vi "LoggingMessageLoop.vi"(8 "Error In":errorcluster, 11 "CommunicationRefs":T1) -> (0 "Error Out":errorcluster)   [LabVIEW 2015]
uses:
  TypeDefs/CommunicationRefs.ctl
  TypeDefs/MessageCluster.ctl
  TypeDefs/FlowData.ctl
  TypeDefs/ClsLastSample.ctl
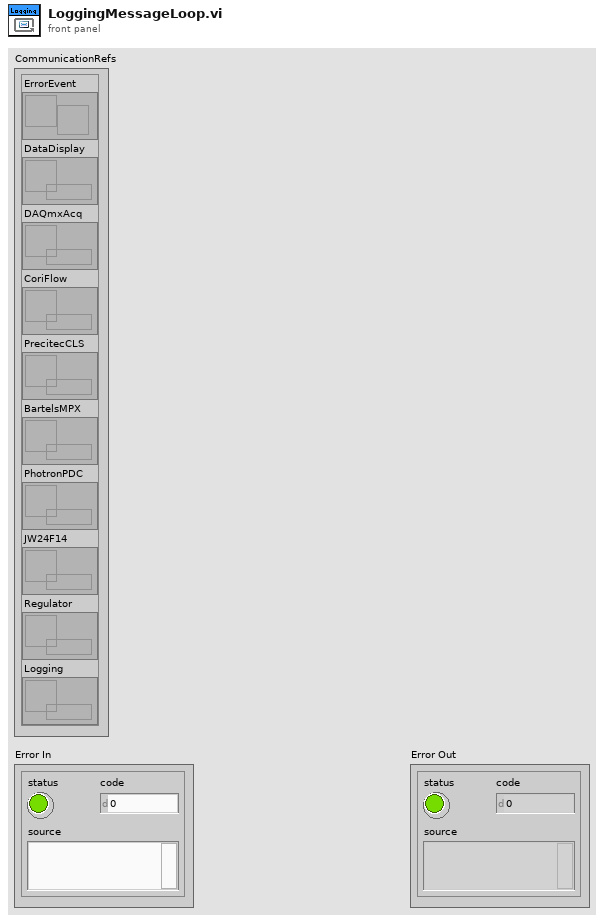
[diagram p1: front panel]
types:
  T1 = typedef "CommunicationRefs.ctl" = cluster{"ErrorEvent":refnum<user-event>, "DataDisplay":refnum<queue>, "DAQmxAcq":refnum<queue>, "CoriFlow":refnum<queue>, "PrecitecCLS":refnum<queue>, "BartelsMPX":refnum<queue>, "PhotronPDC":refnum<queue>, "JW24F14":refnum<queue>, "Regulator":refnum<queue>, "Logging":refnum<queue>}
  T2 = enum16{"open", "open or create", "create or replace", "create", "open (read-only)"}
  T3 = typedef "FlowData.ctl" = cluster{"Setpoint Direct":sgl, "Setpoint Percentage":dbl, "Flow Direct":sgl, "Flow Percentage [%]":dbl, "Fluid Temperature [°C]":sgl, "Fluid Density [kg/m³]":sgl, "Alarm":string}
  T4 = typedef "ClsLastSample.ctl" = cluster{"Global Signals":dbl[], "Peak Signals":dbl[][], "Film Height [µm]":dbl, "standard deviation [µm]":dbl, "variance":dbl}
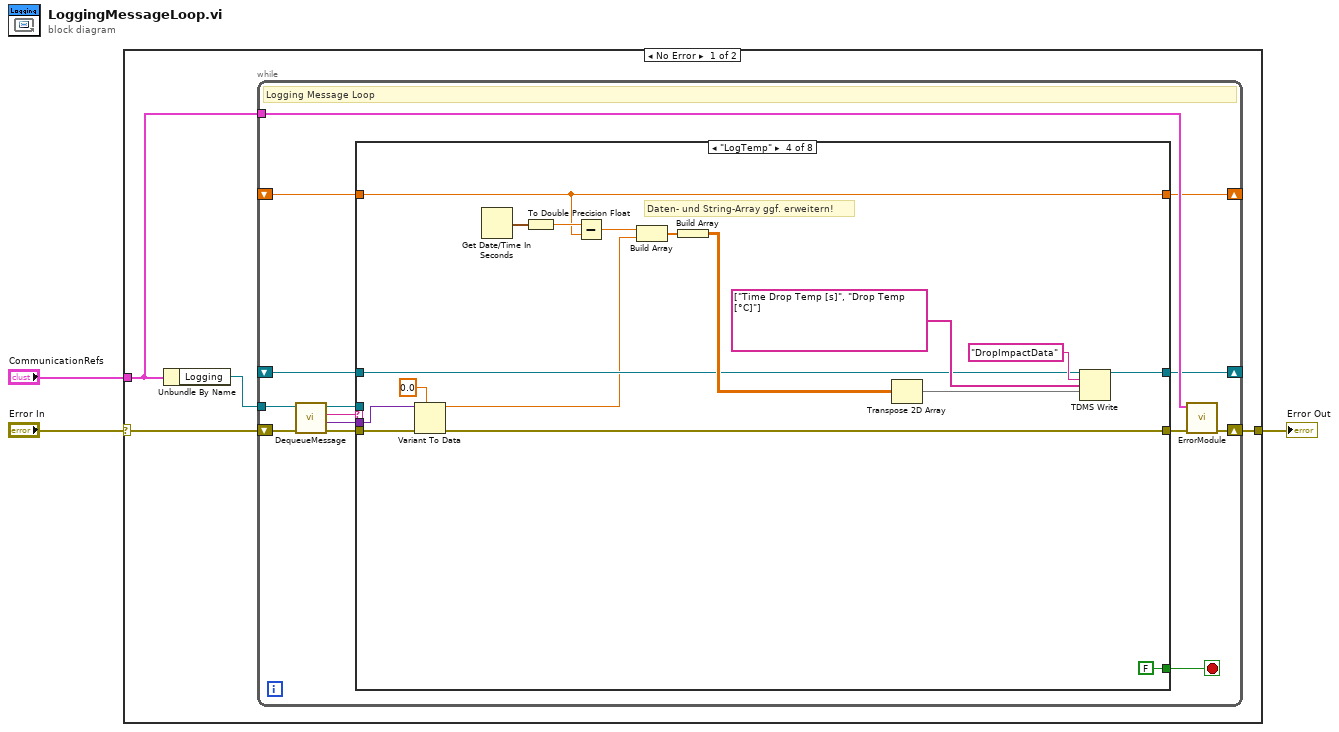
[diagram p0: block diagram]
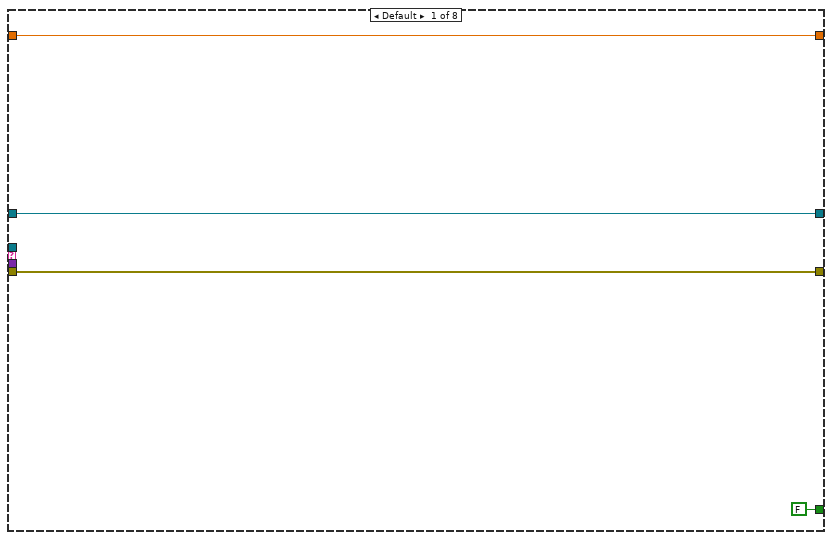
[diagram p2: hidden frame]
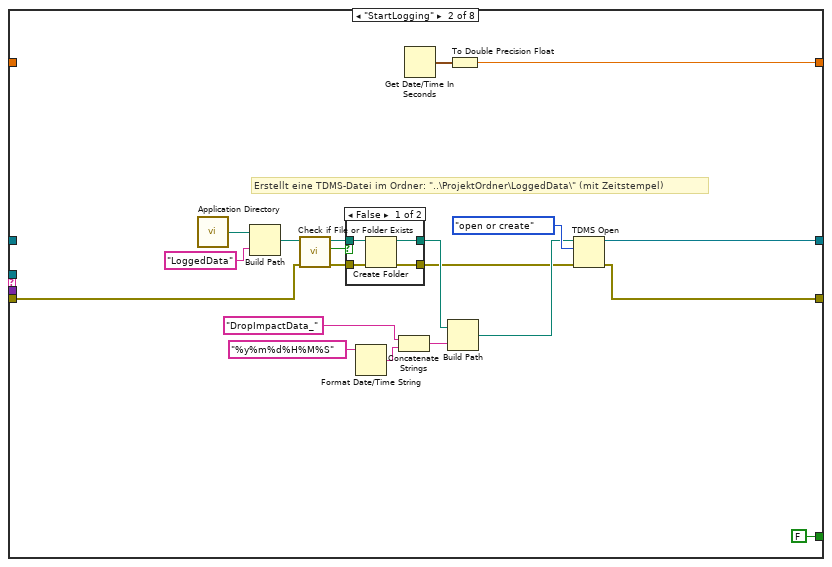
[diagram p3: hidden frame]
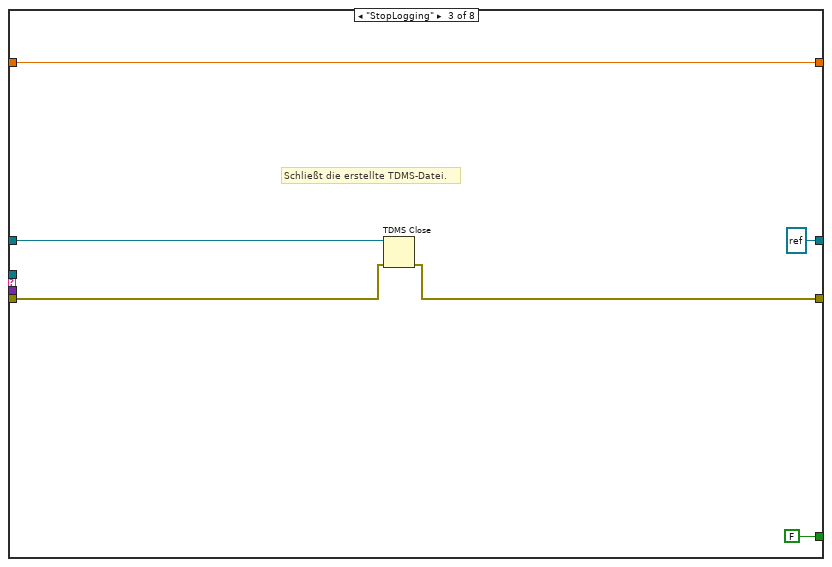
[diagram p5: hidden frame]
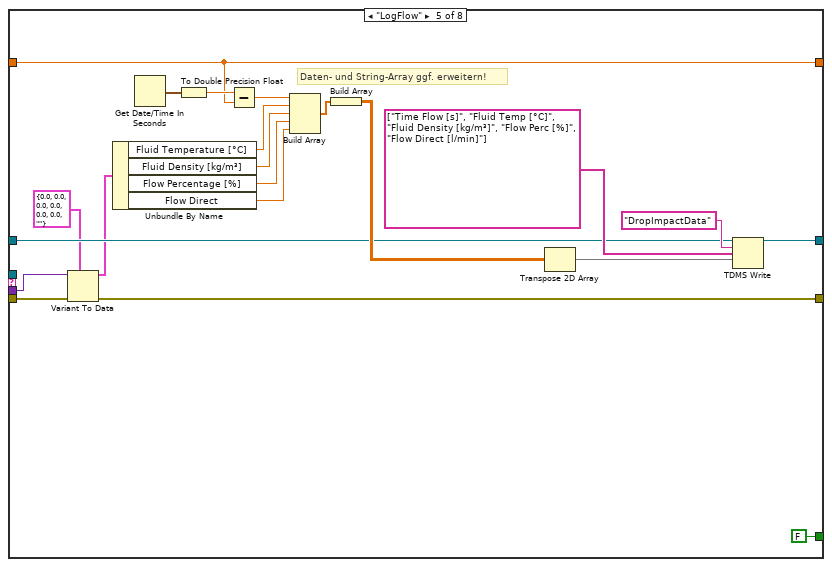
[diagram p6: hidden frame]
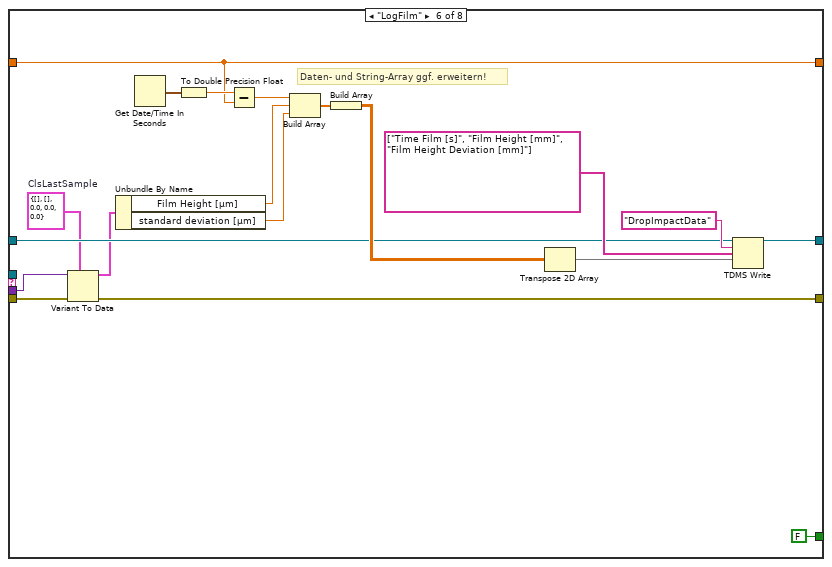
[diagram p7: hidden frame]
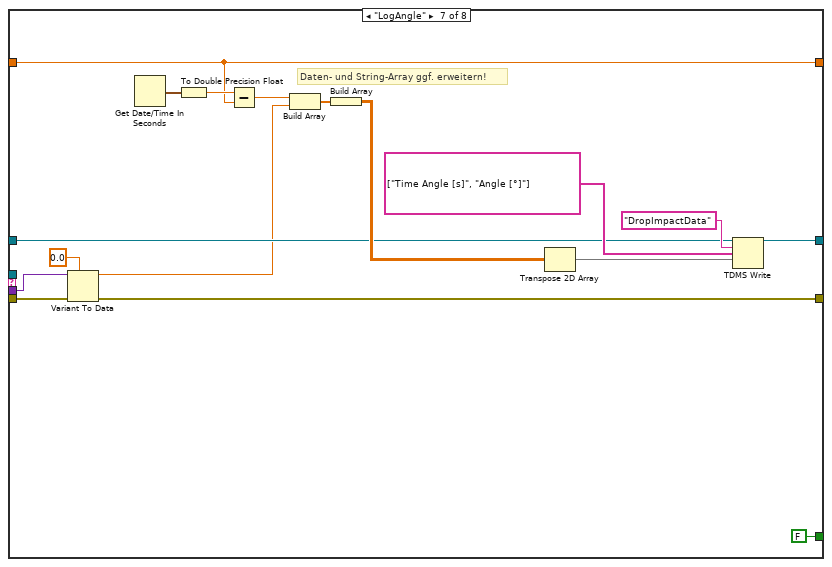
[diagram p8: hidden frame]
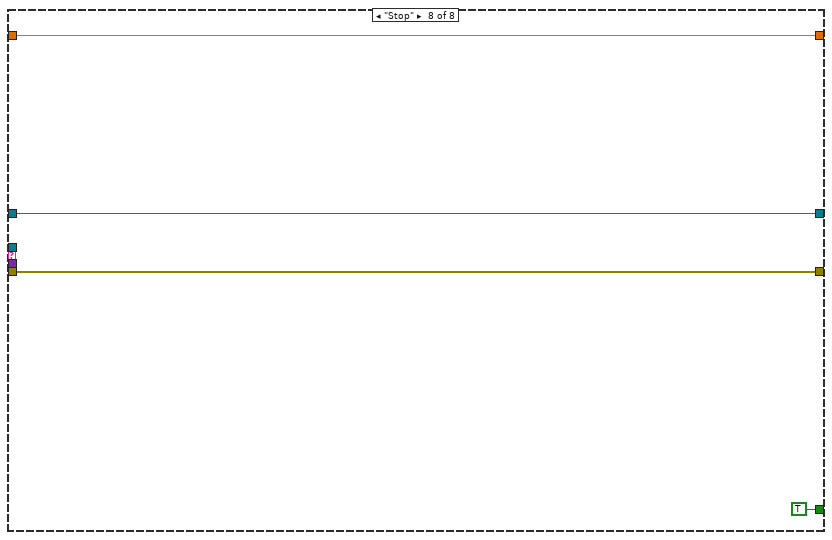
[diagram p9: hidden frame]
diagram:
  n1 = case shown="No Error" "Error In" {
    selector: "Error In" -> [w6 w136]
    tunnel: [w5 w136] -> w2
    tunnel: "CommunicationRefs" -> [w4 _]
    frame No Error {
      n2 = Unbundle By Name(w4) -> ("Logging"=w7:refnum<queue>)
      n3 = while {
        tunnel: w7 -> [w21]
        tunnel: w4 -> [w14]
        shift-right: [w15] -> w5
        shift-left: w6 -> [w20]
        shift-right: [w11] -> _
        shift-left: _ -> [w10]
        shift-right: [w9] -> _
        shift-left: _ -> [w8]
        stop <- w13 stop-if-true
        # "Logging Message Loop"
        n4 = call "DequeueMessage.vi"("error in (no error)"=w20, "MessageQueue"=w21) -> ("error out"=w16:errorcluster, "MessageData"=w17:variant, "Message"=w18:string, "dupMessageQueue"=w19:refnum<queue>)  [unwired: 6 in]
        n5 = case shown="\"LogTemp\"" w18 {
          tunnel: w19 -> [_ _ _ _ _ _ _ _]
          tunnel: w17 -> [_ _ _ w63 w84 w103 w120 _]
          tunnel: w16 -> [w23 w26 w55 w62 w83 w102 w119 w133]
          tunnel: [FALSE FALSE FALSE FALSE FALSE FALSE FALSE TRUE] -> w13
          tunnel: [w23 w29 w54 w58 w75 w96 w115 w133] -> w12
          tunnel: [w24 w28 refnum<k34> refnum ("tdms file out") w64 w85 w104 w121 w132] -> w11
          tunnel: w10 -> [w24 _ w56 w65 w86 w105 w122 w132]
          tunnel: [w25 w27 w52 w61 w82 w101 w118 w134] -> w9
          tunnel: w8 -> [w25 _ w52 w61 w82 w101 w118 w134]
          frame Default {
          }
          frame "StartLogging" {
            # "Erstellt eine TDMS-Datei im Ordner: \"..\\ProjektOrdner\\LoggedData\\\" (mit Zeitstempel)"
            n6 = call <vilib>:"Application Directory.vi"() -> ("Application Directory"=w44:path)
            n7 = Build Path(base path=w44, name or relative path="LoggedData") -> (appended path=w42:path)
            n8 = call <vilib>:"Check if File or Folder Exists.vi"("error in (no error)"=w26, "path"=w42) -> ("error out"=w39:errorcluster, "file or folder exists?"=w41:bool, "dup path"=w40:path)  [unwired: 7 in]
            n9 = case shown="False" w41 {
              tunnel: w40 -> [w49 w51]
              tunnel: [w47 w51] -> w38
              tunnel: [w46 w50] -> w30
              tunnel: w39 -> [w48 w50]
              frame False {
                n10 = Create Folder(path (use dialog)=w49, error in=w48) -> (created path=w47:path, error out=w46:errorcluster)  [unwired: 1 in, 1 out]
              }
              frame True {
              }
            }
            n11 = Format Date/Time String(time format string (%c)="%y%m%d%H%M%S") -> (date/time string=w35:string)  [unwired: 2 in]
            n12 = Concatenate Strings("DropImpactData_" ("string"), w35) -> (w33:string)
            n13 = Get Date/Time In Seconds() -> (seconds since 1Jan1904=w37:timestamp)
            n14 = Build Path(base path=w38, name or relative path=w33) -> (appended path=w31:path)
            n15 = To Double Precision Float(number=w37) -> (double precision float=w27:dbl)
            n16 = TDMS Open(8:w30, 10:T2."open or create" ("operation (0:open)"), 11:w31) -> (0:w29:errorcluster, 3:w28:refnum<k34>)  [unwired: 4 in]
          }
          frame "StopLogging" {
            # "Schließt die erstellte TDMS-Datei."
            n17 = TDMS Close(8:w55, 11:w56) -> (0:w54:errorcluster)  [unwired: 1 out]
          }
          frame "LogTemp" {
            # "Daten- und String-Array ggf. erweitern!"
            n18 = Variant To Data(error in=w62, type=0.0, Variant=w63) -> (data=w59:dbl, error out=w58:errorcluster)
            n19 = Get Date/Time In Seconds() -> (seconds since 1Jan1904=w72:timestamp)
            n20 = To Double Precision Float(number=w72) -> (double precision float=w71:dbl)
            n21 = Subtract(x=w71, y=w61) -> (x-y=w70:dbl)
            n22 = Build Array(w70, w59) -> (w69:dbl[])
            n23 = Build Array(w69) -> (w67:dbl[][])
            n24 = Transpose 2D Array(2D array=w67) -> (transposed array=w66:dbl[][])
            n25 = TDMS Write(0:w65, 5:"DropImpactData" ("group name in (Untitled)"), 7:string[] ["Time Drop Temp [s]", "Drop Temp [°C]"], 9:w66) -> (4:w64:refnum<k34>)  [unwired: 2 in, 3 out]
          }
          frame "LogFlow" {
            # "Daten- und String-Array ggf. erweitern!"
            n26 = Variant To Data(error in=w83, type=T3 {"Setpoint Direct"=0.0, "Setpoint Percentage"=0.0, "Flow Direct"=0.0, "Flow Percentage [%]"=0.0, "Fluid Temperature [°C]"=0.0, "Fluid Density [kg/m³]"=0.0, "Alarm"=""} ("Sensor Data"), Variant=w84) -> (data=w80:T3, error out=w75:errorcluster)
            n27 = Unbundle By Name(w80) -> ("Fluid Temperature [°C]"=w79:sgl, "Fluid Density [kg/m³]"=w78:sgl, "Flow Percentage [%]"=w77:dbl, "Flow Direct"=w76:sgl)
            n28 = Get Date/Time In Seconds() -> (seconds since 1Jan1904=w93:timestamp)
            n29 = To Double Precision Float(number=w93) -> (double precision float=w92:dbl)
            n30 = Subtract(x=w92, y=w82) -> (x-y=w91:dbl)
            n31 = Build Array(w91, w79, w78, w77, w76) -> (w90:dbl[])
            n32 = Build Array(w90) -> (w88:dbl[][])
            n33 = Transpose 2D Array(2D array=w88) -> (transposed array=w87:dbl[][])
            n34 = TDMS Write(0:w86, 5:"DropImpactData" ("group name in (Untitled)"), 7:string[] ["Time Flow [s]", "Fluid Temp [°C]", "Fluid Density [kg/m³]", "Flow Perc [%]", "Flow Direct [l/min]"], 9:w87) -> (4:w85:refnum<k34>)  [unwired: 2 in, 3 out]
          }
          frame "LogFilm" {
            w100 = T4 {"Global Signals"=[], "Peak Signals"=[], "Film Height [µm]"=0.0, "standard deviation [µm]"=0.0, "variance"=0.0}  # ClsLastSample
            # "Daten- und String-Array ggf. erweitern!"
            n35 = Variant To Data(error in=w102, type=w100, Variant=w103) -> (data=w99:T4, error out=w96:errorcluster)
            n36 = Unbundle By Name(w99) -> ("Film Height [µm]"=w98:dbl, "standard deviation [µm]"=w97:dbl)
            n37 = Get Date/Time In Seconds() -> (seconds since 1Jan1904=w112:timestamp)
            n38 = To Double Precision Float(number=w112) -> (double precision float=w111:dbl)
            n39 = Subtract(x=w111, y=w101) -> (x-y=w110:dbl)
            n40 = Build Array(w110, w98, w97) -> (w109:dbl[])
            n41 = Build Array(w109) -> (w107:dbl[][])
            n42 = Transpose 2D Array(2D array=w107) -> (transposed array=w106:dbl[][])
            n43 = TDMS Write(0:w105, 5:"DropImpactData" ("group name in (Untitled)"), 7:string[] ["Time Film [s]", "Film Height [mm]", "Film Height Deviation [mm]"], 9:w106) -> (4:w104:refnum<k34>)  [unwired: 2 in, 3 out]
          }
          frame "LogAngle" {
            # "Daten- und String-Array ggf. erweitern!"
            n44 = Variant To Data(error in=w119, type=0.0, Variant=w120) -> (data=w117:dbl, error out=w115:errorcluster)
            n45 = Get Date/Time In Seconds() -> (seconds since 1Jan1904=w129:timestamp)
            n46 = To Double Precision Float(number=w129) -> (double precision float=w128:dbl)
            n47 = Subtract(x=w128, y=w118) -> (x-y=w127:dbl)
            n48 = Build Array(w127, w117) -> (w126:dbl[])
            n49 = Build Array(w126) -> (w124:dbl[][])
            n50 = Transpose 2D Array(2D array=w124) -> (transposed array=w123:dbl[][])
            n51 = TDMS Write(0:w122, 5:"DropImpactData" ("group name in (Untitled)"), 7:string[] ["Time Angle [s]", "Angle [°]"], 9:w123) -> (4:w121:refnum<k34>)  [unwired: 2 in, 3 out]
          }
          frame "Stop" {
          }
        }
        n52 = call "ErrorModule.vi"("Error In"=w12, "CommunicationRefs"=w14) -> ("Error Out"=w15:errorcluster)  [unwired: 9 in]
      }
    }
    frame Error {
    }
  }
  "Error Out" <- w2
